vi "Main.vi"() -> ()   [LabVIEW 2019]
doc: "使用该模板构建简单状态机设计模式。各状态执行代码并决定转移状态。"
uses:
  controls/State.ctl
  <vilib>/imath/engines/lvmath/Deprecated/data.ctl
  <vilib>/DAQmx/read.llb/DAQmx Read (Digital 1D Bool 1Chan 1Samp).vi
  <vilib>/DAQmx/create/channels.llb/DAQmx Create Channel (DI-Digital Input).vi
panel:
  in  "数据保存":bool
  out "数字":u32
  out "7":bool
  out "6":bool
  out "5":bool
  out "4":bool
  out "3":bool
  out "2":bool
  out "1":bool
  out "触发信息":string
  out "error out":errorcluster caption="错误输出"
  in  "停止":bool
  in  "停止测试":bool
  in  "开始测试":bool
  in  "退出":bool
  # "先停止测试再保存数据"
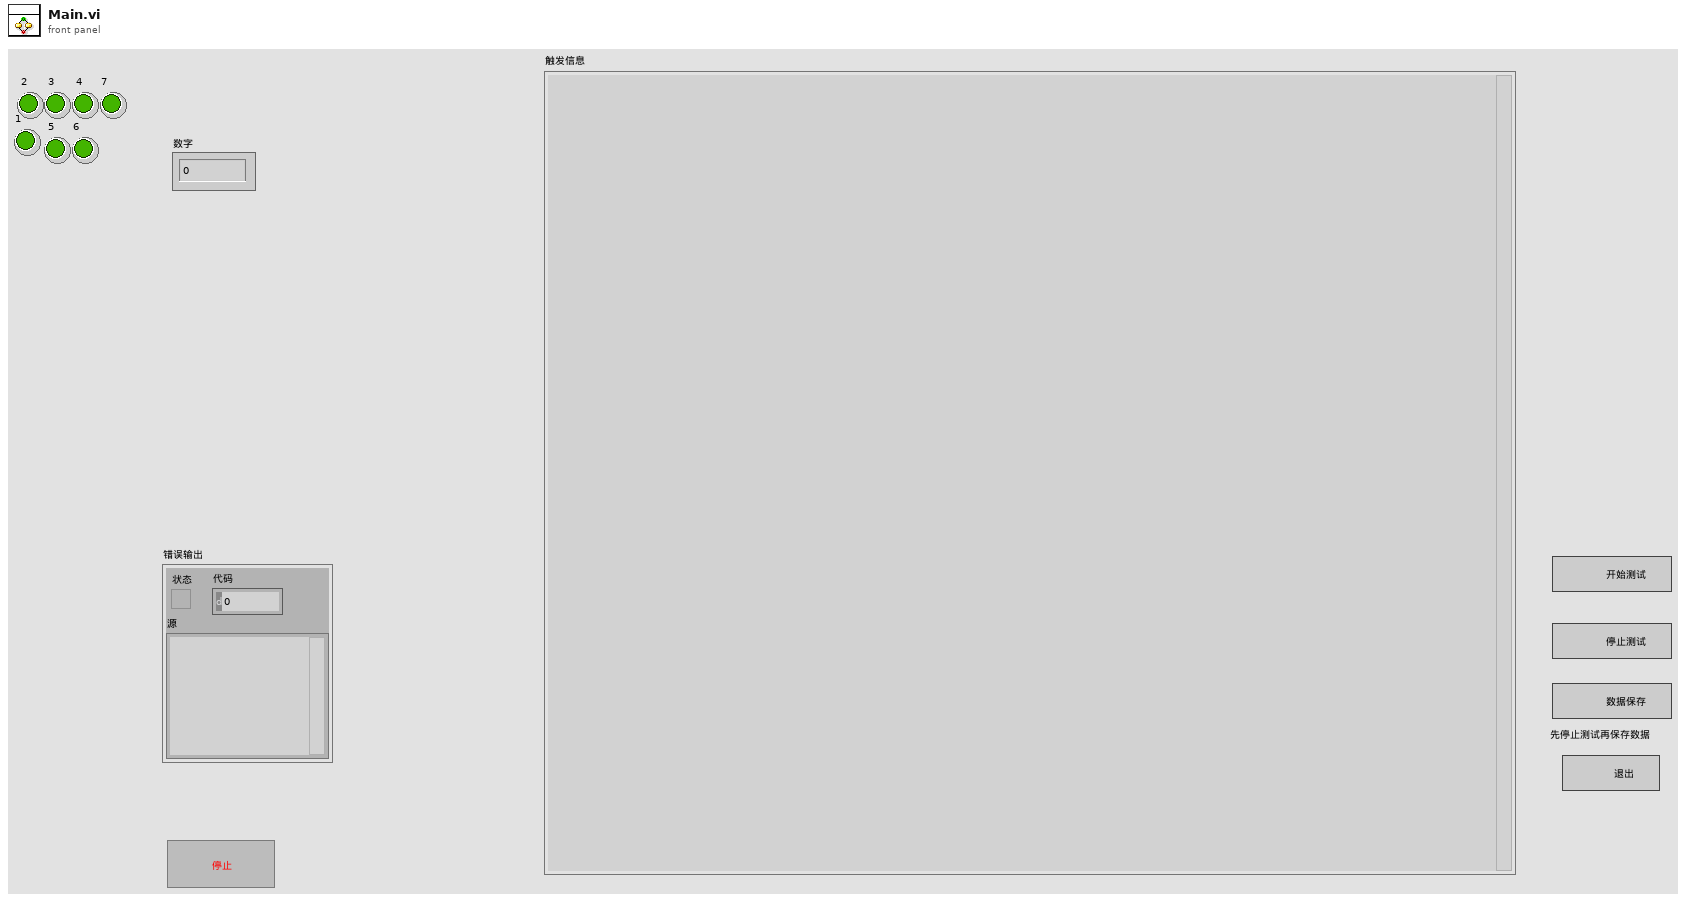
[diagram p1: front panel]
types:
  T1 = typedef "data.ctl" = dbl
  T2 = typedef "State.ctl" = enum16{"Initialize", "Wait for Event", "开始测试", "数据保存", "触发状态记录", "Exit"}
  T3 = enum16{"open", "replace", "create", "open or create", "replace or create", "replace or create with confirmation"}
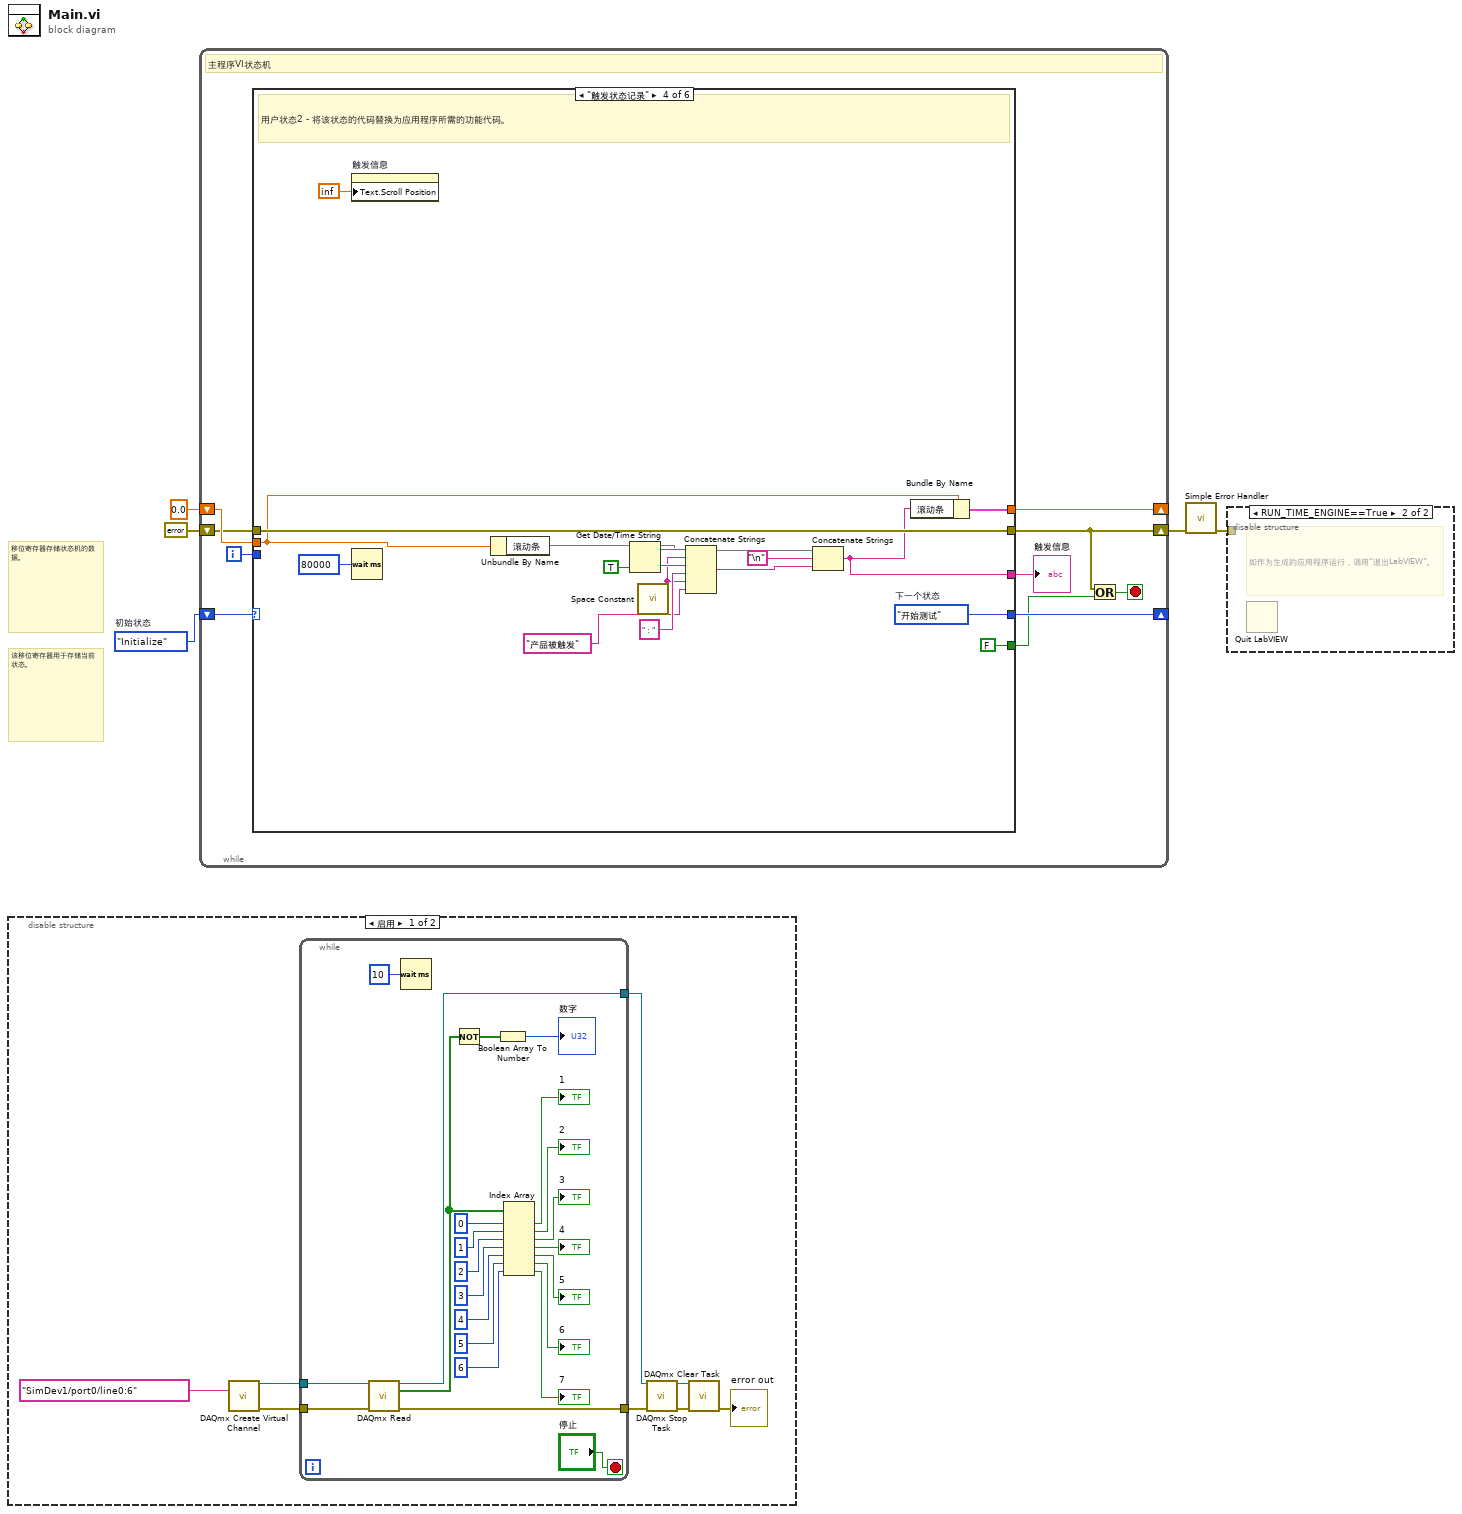
[diagram p0: block diagram]
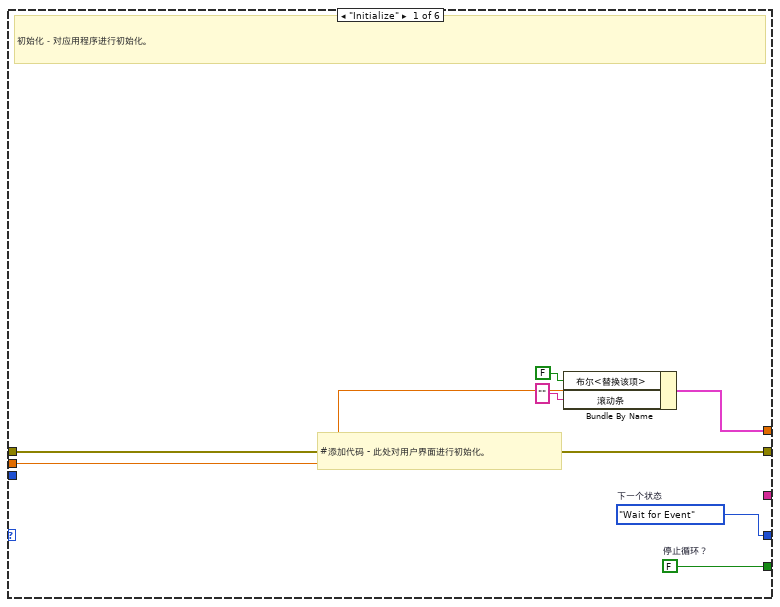
[diagram p4: hidden frame]
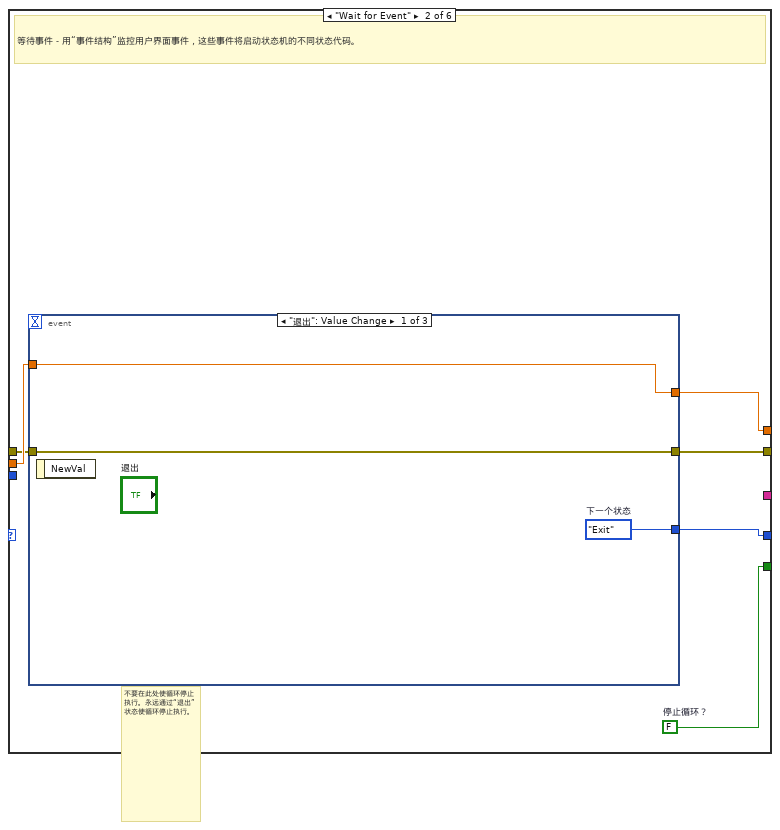
[diagram p5: hidden frame]
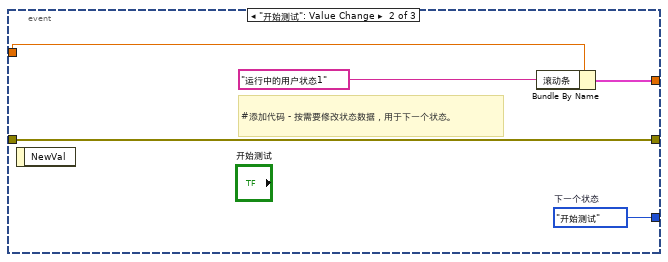
[diagram p6: hidden frame]
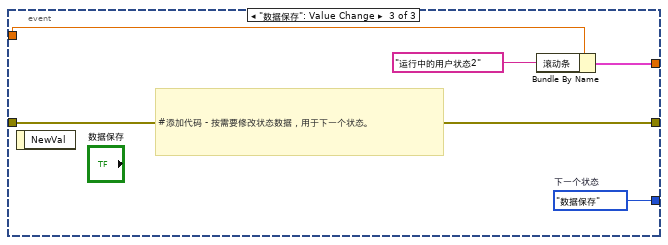
[diagram p7: hidden frame]
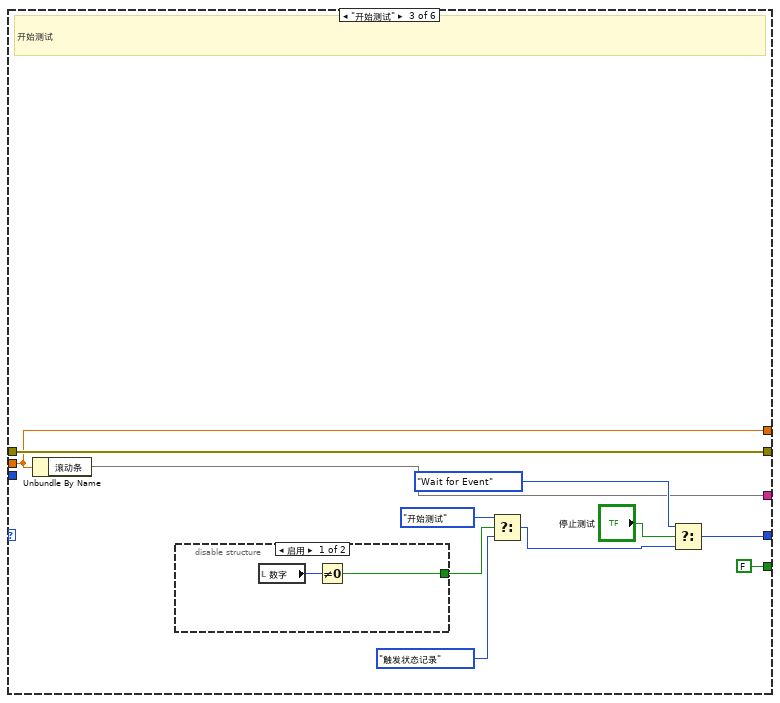
[diagram p8: hidden frame]
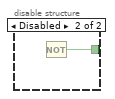
[diagram p9: hidden frame]
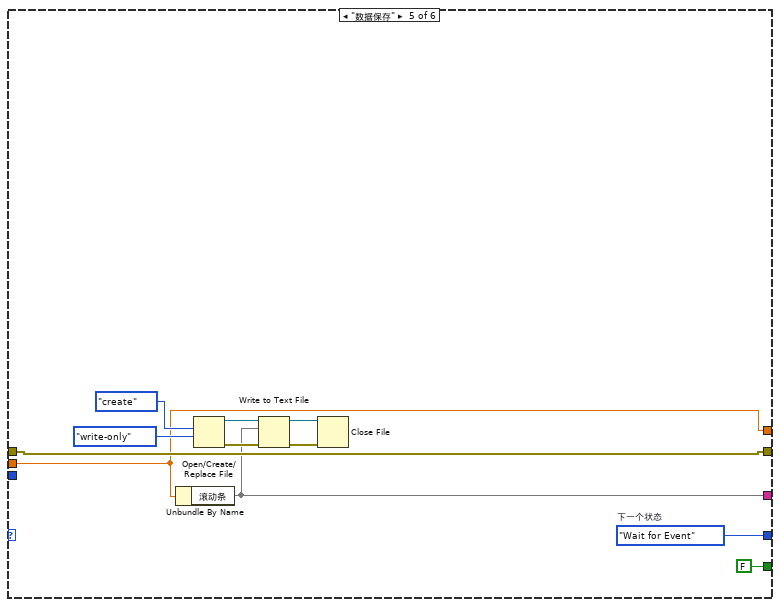
[diagram p10: hidden frame]
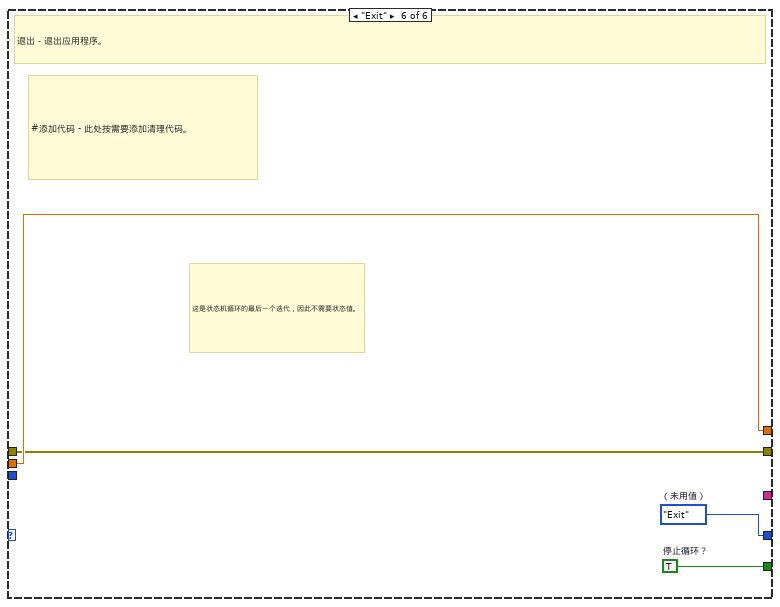
[diagram p11: hidden frame]
diagram:
  w5 = State."Initialize"  # 初始状态
  # "移位寄存器存储状态机的数据。"
  # "该移位寄存器用于存储当前状态。"
  n1 = disable-structure shown="启用" {
    frame Enabled {
      n2 = call-poly <vilib>:"DAQmx Create Virtual Channel.vi"("lines"=tag "SimDev1/port0/line0:6") -> ("task out"=w12:refnum<k21>, "error out"=w11:errorcluster)  [unwired: 13 in]
      n3 = while {
        tunnel: w12 -> [w36]
        tunnel: w11 -> [w35]
        tunnel: [w34] -> w10
        tunnel: [w33] -> w9
        stop <- "停止" stop-if-true
        n4 = call-poly <vilib>:"DAQmx Read.vi"("task/channels in"=w36, "error in"=w35) -> ("task out"=w34:refnum<k21>, "data"=w15:bool[], "error out"=w33:errorcluster)  [unwired: 11 in]
        n5 = Wait (ms)(milliseconds to wait=u32 10 ("等待时间（毫秒）")) -> ()  [unwired: 1 out]
        n6 = Not(x=w15) -> (.not. x?=w14:bool[])
        n7 = Boolean Array To Number(Boolean array=w14) -> (number=→"数字":u32)
        n8 = Index Array(array=w15, index #1=0 ("索引"), index #2=1 ("索引"), index #3=2 ("索引"), index #4=3 ("索引"), index #5=4 ("索引"), index #6=5 ("索引"), index #7=6 ("索引")) -> (element #1=→"1":bool, element #2=→"2":bool, element #3=→"3":bool, element #4=→"4":bool, element #5=→"5":bool, element #6=→"6":bool, element #7=→"7":bool)
      }
      n9 = call <vilib>:"DAQmx Stop Task.vi"("task/channels in"=w10, "error in"=w9) -> ("task out"=w7:refnum<k21>, "error out"=w8:errorcluster)  [unwired: 12 in]
      n10 = call <vilib>:"DAQmx Clear Task.vi"("task in"=w7, "error in"=w8) -> ("error out"=→"error out":errorcluster)  [unwired: 13 in]
    }
    frame Disabled {
    }
  }
  n11 = while {
    shift-right: [w45] -> _
    shift-left: w5 -> [w46]
    shift-right: [w43] -> _
    shift-left: T1 0.0 ("Data") -> [w44]
    shift-right: [w39] -> w2
    shift-left: errorcluster {"status"=FALSE, "code"=0, "source"=""} ("error constant") -> [w42]
    i -> [w38]
    stop <- w40 stop-if-true
    # "主程序VI状态机"
    n12 = case shown="\"触发状态记录\"" w46 {
      tunnel: [w53 w59 w80 w104 w114 w119] -> w45
      tunnel: [w52 w58 FALSE ("Stop Loop?") FALSE ("Stop Loop?") FALSE ("Stop Loop?") w117] -> w41
      tunnel: w44 -> [w51 w57 w74 w90 w109 w118]
      tunnel: [w50 w56 w74 w89 w109 w118] -> w43
      tunnel: w42 -> [w48 w55 w82 w102 w115 w116]
      tunnel: [w48 w54 w82 w102 w115 w116] -> w39
      tunnel: w38 -> [_ _ _ _ _ _]
      tunnel: [_ _ w73 w92 w105 _] -> w37
      frame "Initialize" {
        w52 = FALSE  # 停止循环？
        w53 = State."Wait for Event"  # 下一个状态
        # "#添加代码 - 此处对用户界面进行初始化。"
        # "初始化－对应用程序进行初始化。"
        n13 = Bundle By Name(cluster=w51, "布尔<替换该项>"=FALSE ("Replace_Me_Boolean"), "滚动条"="") -> (w50:cluster{})
      }
      frame "Wait for Event" {
        w58 = FALSE  # 停止循环？
        # "不要在此处使循环停止执行。永远通过“退出”状态使循环停止执行。"
        # "等待事件－用“事件结构”监控用户界面事件，这些事件将启动状态机的不同状态代码。"
        n14 = event shown="[0] \"退出\": Value Change" {
          selector: _ -> [_ _ _]
          dyn-events: _ -> [_ _ _]
          timeout: _ -> [_ _ _]
          tunnel: [w62 w67 w72] -> w59
          tunnel: w57 -> [w61 w66 w71]
          tunnel: [w61 w65 w70] -> w56
          tunnel: w55 -> [w60 w63 w68]
          tunnel: [w60 w63 w68] -> w54
          event "退出": Value Change {
            w62 = State."Exit"  # 下一个状态
            n15 = event-data() -> ()  [unwired: 1 in, 1 out]
          }
          event "开始测试": Value Change {
            w67 = State."开始测试"  # 下一个状态
            # "#添加代码 - 按需要修改状态数据，用于下一个状态。"
            n16 = event-data() -> ()  [unwired: 1 in, 1 out]
            n17 = Bundle By Name(cluster=w66, "滚动条"="运行中的用户状态1" ("Running User State 1")) -> (w65:cluster{})
          }
          event "数据保存": Value Change {
            w72 = State."数据保存"  # 下一个状态
            # "#添加代码 - 按需要修改状态数据，用于下一个状态。"
            n18 = event-data() -> ()  [unwired: 1 in, 1 out]
            n19 = Bundle By Name(cluster=w71, "滚动条"="运行中的用户状态2" ("Running User State 2")) -> (w70:cluster{})
          }
        }
      }
      frame "开始测试" {
        # "开始测试"
        n20 = Unbundle By Name(w74) -> ("滚动条"=w73)
        n21 = disable-structure shown="启用" {
          disable-tunnel: [w84 w86] -> w75
          frame Enabled {
            n22 = local read "数字"() -> (w85:u32)
            n23 = Not Equal To 0?(x=w85) -> (x != 0?=w84:bool)
          }
          frame Disabled {
            n24 = Not() -> (x=w87:bool, .not. x?=w86:bool)
          }
        }
        n25 = Select(t=State."开始测试" ("下一个状态"), s=w75, f=State."触发状态记录" ("下一个状态")) -> (s? t:f=w76:T2)
        n26 = Select(t=State."Wait for Event" ("下一个状态"), s="停止测试", f=w76) -> (s? t:f=w80:T2)
      }
      frame "触发状态记录" {
        w104 = State."开始测试"  # 下一个状态
        # "用户状态2 - 将该状态的代码替换为应用程序所需的功能代码。"
        n27 = property on="触发信息" class="Str"("Text.Scroll Position"=inf) -> ()  [unwired: 2 in, 2 out]
        n28 = Wait (ms)(milliseconds to wait=u32 80000 ("等待时间（毫秒）")) -> ()  [unwired: 1 out]
        n29 = Unbundle By Name(w90) -> ("滚动条"=w98)
        n30 = Get Date/Time String(want seconds? (F)=TRUE ("需要秒？(F)")) -> (date string=w100:string, time string=w99:string)  [unwired: 2 in]
        n31 = call <vilib>:"Space Constant.vi"() -> ("String"=w95:string)
        n32 = Concatenate Strings(w100, w95, w99, "：" ("字符串"), w95, "产品被触发" ("字符串")) -> (w93:string)
        n33 = Concatenate Strings(w98, "\n", w93) -> (w92:string)
        n34 = Bundle By Name(cluster=w90, "滚动条"=w92) -> (w89:cluster{})
      }
      frame "数据保存" {
        w114 = State."Wait for Event"  # 下一个状态
        n35 = Unbundle By Name(w109) -> ("滚动条"=w105)
        n36 = Open/Create/Replace File(operation (0:open)=T3."create" ("操作(0:open)"), access (0:read/write)=enum16{"read/write", "read-only", "write-only"}."write-only" ("权限(0:read/write)")) -> (refnum out=w110:refnum<file>, error out=w108:errorcluster)  [unwired: 4 in, 1 out]
        n37 = Write to Text File(file (use dialog)=w110, text=w105, error in=w108) -> (refnum out=w107:refnum<file>, error out=w106:errorcluster)  [unwired: 1 in, 1 out]
        n38 = Close File(refnum=w107, error in=w106) -> ()  [unwired: 2 out]
      }
      frame "Exit" {
        w117 = TRUE  # 停止循环？
        w119 = State."Exit"  # （未用值）
        # "#添加代码 - 此处按需要添加清理代码。"
        # "这是状态机循环的最后一个迭代，因此不需要状态值。"
        # "退出－退出应用程序。"
      }
    }
    "触发信息" <- w37
    n39 = Or(x=w39, y=w41) -> (x .or. y?=w40:bool)
  }
  n40 = call <vilib>:"Simple Error Handler.vi"("error in (no error)"=w2) -> ("error out"=w1:errorcluster)  [unwired: 4 in, 4 out]
  n41 = disable-structure shown="RUN_TIME_ENGINE==True" {
    disable-tunnel: w1 -> [_ _]
    frame condition #0 (active) {
    }
    frame condition #1 {
      # "如作为生成的应用程序运行，调用“退出LabVIEW”。"
      n42 = Quit LabVIEW() -> ()  [unwired: 1 in]
    }
  }
